vi "Route Editor.vi"(10 "Image In":T1, 11 "Image Path":path=path "D:/Dropbox (Testview)/Shared Projects/BELKIN Laser - R&D/Software/DEMO Code/Images/Vlad Color 3.png") -> (2 "Image":T1(plugin-control))   [LabVIEW 2015]
uses:
  <vilib>/vision/Image Controls.llb/IMAQ Image.ctl
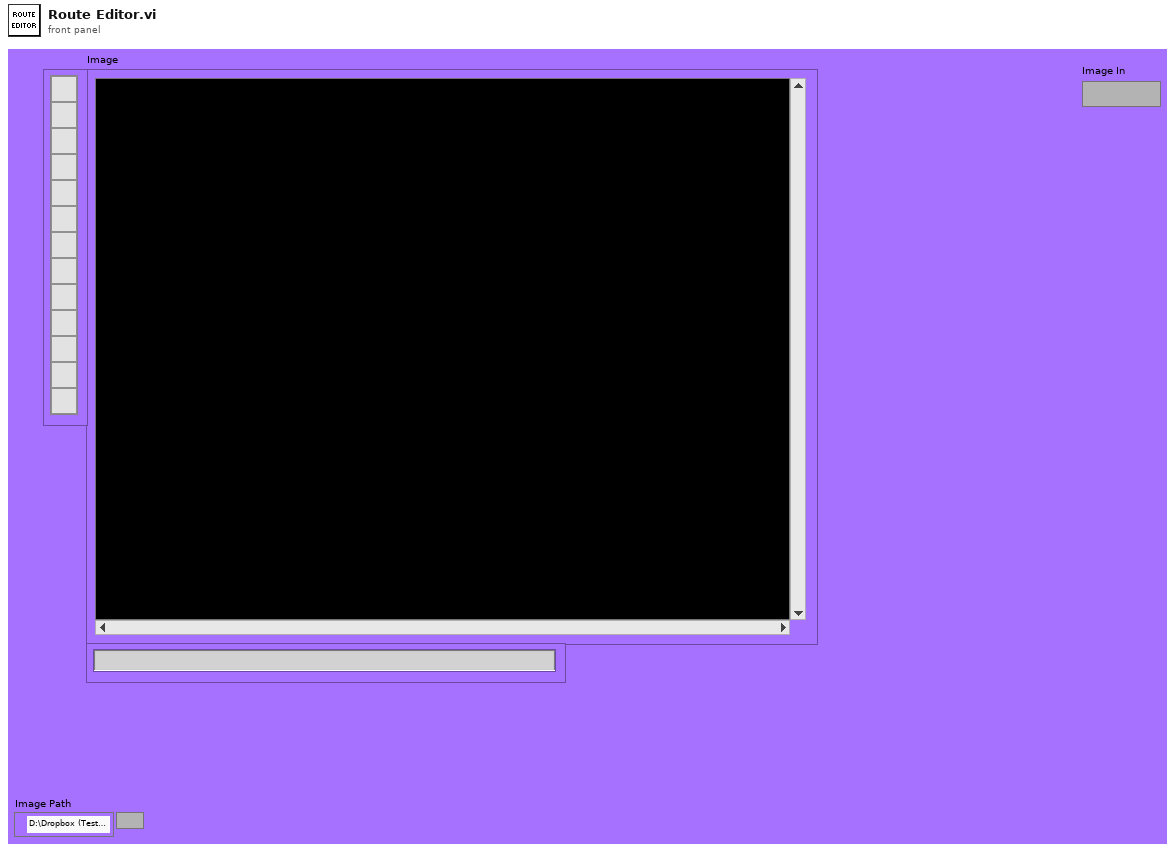
[diagram p1: front panel]
types:
  T1 = typedef "IMAQ Image.ctl" = refnum<image>
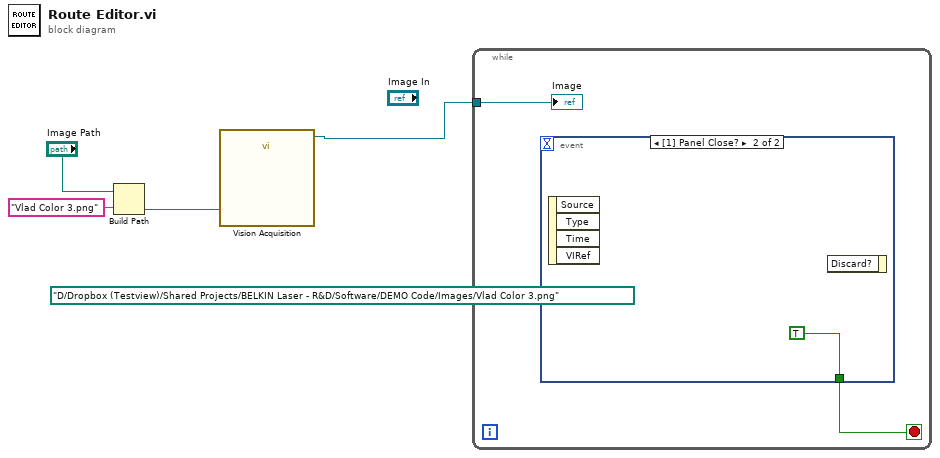
[diagram p0: block diagram]
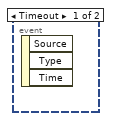
[diagram p2: hidden frame]
diagram:
  (unwired) path "D:/Dropbox (Testview)/Shared Projects/BELKIN Laser - R&D/Software/DEMO Code/Images/Vlad Color 3.png" ("Image Path")
  n1 = Build Path(base path="Image Path", name or relative path="Vlad Color 3.png") -> (appended path=w1:path)
  n2 = call "Vision Acquisition"("Image Path"=w1) -> ("Image Out"=w4:T1)  [unwired: 25 in, 1 out]
  n3 = while {
    tunnel: w4 -> [w6]
    stop <- w5 stop-if-true
    n4 = event shown="[1] Panel Close?" {
      selector: _ -> [_ _]
      dyn-events: _ -> [_ _]
      timeout: _ -> [_ _]
      tunnel: [_ TRUE] -> w5
      event Timeout {
        n5 = event-data() -> ()  [unwired: 1 in, 3 out]
      }
      event Panel Close? {
        n6 = event-data() -> ()  [unwired: 1 in, 4 out]
        n7 = event-data() -> ()  [unwired: 2 in, 1 out]
      }
    }
    "Image" <- w6
  }
